vi "Stop.vi"(8 "error in (no error)":errorcluster, 11 "Control in":refnum<class "Control-Server.lvclass">) -> (0 "error out":errorcluster, 3 "Control out":refnum<class "Control-Server.lvclass">)   [LabVIEW 2020, in "Control-Server.lvclass"]
uses:
  Control-Server.lvclass
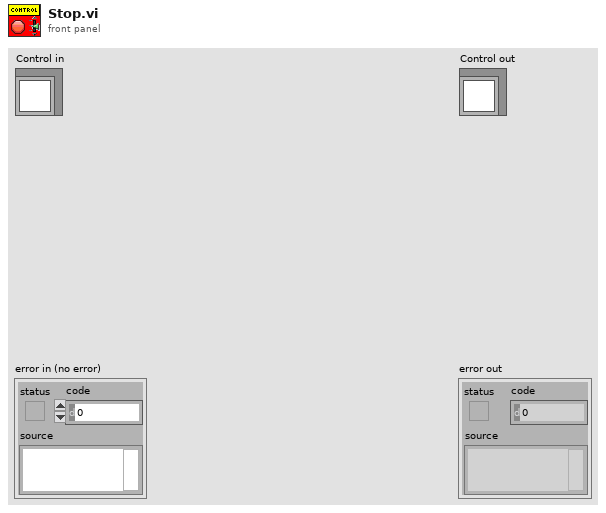
[diagram p1: front panel]
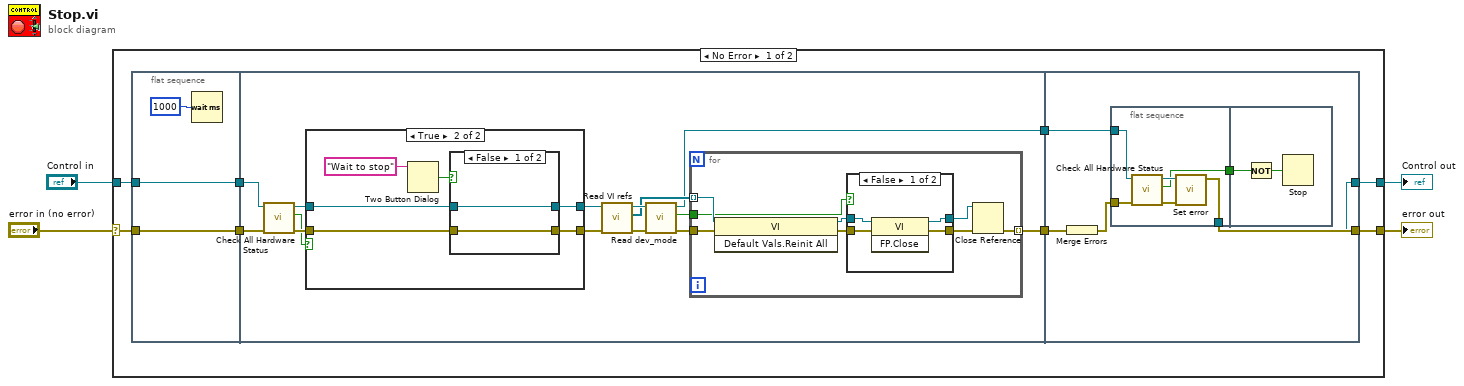
[diagram p0: block diagram]
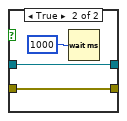
[diagram p3: hidden frame]
diagram:
  n1 = case shown="No Error" "error in (no error)" {
    selector: "error in (no error)" -> [w5 w73]
    tunnel: [w10 w73] -> w3
    tunnel: [w9 w72] -> w1
    tunnel: "Control in" -> [w8 w72]
    frame No Error {
      n2 = flat-sequence {
        tunnel: w8 -> [w14]
        tunnel: [w14] -> w7
        tunnel: [w13] -> w6
        tunnel: w5 -> [w13]
        tunnel: [w22] -> w12
        tunnel: [w21] -> w11
        tunnel: w7 -> [w20]
        tunnel: w6 -> [w17]
        tunnel: w12 -> [w61]
        tunnel: w11 -> [w62]
        tunnel: [w58] -> w10
        tunnel: [w57] -> w9
        frame #0 {
          n3 = Wait (ms)(milliseconds to wait=u32 1000 ("attente (ms)")) -> ()  [unwired: 1 out]
        }
        frame #1 {
          n4 = call "Check All Hardware Status.vi"("error in (no error)"=w17, "Control en entrée"=w20) -> ("error out"=w18:errorcluster, "HARDWARE"=w16:bool, "Control en sortie"=w19:refnum<class "Control-Server.lvclass">)  [unwired: 7 in]
          n5 = case shown="True" w16 {
            tunnel: [w31 w35] -> w24
            tunnel: [w30 w33] -> w23
            tunnel: w19 -> [w31 w34]
            tunnel: w18 -> [w30 w32]
            frame False {
            }
            frame True {
              n6 = Two Button Dialog(message="Wait to stop") -> (T button?=w36:bool)  [unwired: 2 in]
              n7 = case shown="False" w36 {
                tunnel: [w39 w41] -> w35
                tunnel: w34 -> [w39 w41]
                tunnel: [w38 w40] -> w33
                tunnel: w32 -> [w38 w40]
                frame False {
                }
                frame True {
                  n8 = Wait (ms)(milliseconds to wait=u32 1000 ("attente (ms)")) -> ()  [unwired: 1 out]
                }
              }
            }
          }
          n9 = call-dynamic "Read VI refs.vi"("error in (no error)"=w23, "Control in"=w24) -> ("error out"=w28:errorcluster, "VI refs"=w25:refnum<vi>[], "Control out"=w27:refnum<class "Control-Server.lvclass">)  [unwired: 7 in]
          n10 = call-dynamic "Read dev_mode.vi"("error in (no error)"=w28, "Control in"=w27) -> ("error out"=w29:errorcluster, "dev_mode"=w26:bool, "Control out"=w21:refnum<class "Control-Server.lvclass">)  [unwired: 7 in]
          n11 = for {
            tunnel: w29 -> [w47]
            tunnel: w25 -> [w50] mode=indexing
            tunnel: [w44] -> w22 mode=indexing
            tunnel: w26 -> [w43]
            n12 = invoke class="VI" method="Default Vals.Reinit All"(reference=w50, error in=w47) -> (reference out=w49:refnum<vi>, error out=w48:errorcluster)  [unwired: 1 in, 1 out]
            n13 = case shown="False" w43 {
              tunnel: w49 -> [w54 w56]
              tunnel: w48 -> [w53 w55]
              tunnel: [w52 w56] -> w46
              tunnel: [w51 w55] -> w45
              frame False {
                n14 = invoke class="VI" method="FP.Close"(reference=w54, error in=w53) -> (reference out=w52:refnum<vi>, error out=w51:errorcluster)  [unwired: 1 in, 1 out]
              }
              frame True {
              }
            }
            n15 = Close Reference(reference=w46, error in (no error)=w45) -> (error out=w44:errorcluster)
          }
        }
        frame #2 {
          n16 = Merge Errors(w61) -> (w60:errorcluster)
          n17 = flat-sequence {
            tunnel: w62 -> [w69]
            tunnel: w60 -> [w68]
            tunnel: [w63] -> w59
            tunnel: [w65] -> w58
            tunnel: [w64] -> w57
            tunnel: w59 -> [w71]
            frame #0 {
              n18 = call "Check All Hardware Status.vi"("error in (no error)"=w68, "Control en entrée"=w69) -> ("error out"=w66:errorcluster, "HARDWARE"=w63:bool, "Control en sortie"=w67:refnum<class "Control-Server.lvclass">)  [unwired: 7 in]
              n19 = call "Set error.vi"("error in (no error)"=w66, "Control-Server in"=w67) -> ("error out"=w65:errorcluster, "Control-Server out"=w64:refnum<class "Control-Server.lvclass">)  [unwired: 8 in]
            }
            frame #1 {
              n20 = Not(x=w71) -> (.not. x?=w70:bool)
              n21 = Stop(stop? (T)=w70) -> ()
            }
          }
        }
      }
    }
    frame Error {
    }
  }
  "error out" <- w3
  "Control out" <- w1
